vi "Remove Server.vi"(8 "error in (no error)":errorcluster, 10 "id":i32, 11 "Variant in":variant) -> (0 "error out":errorcluster, 3 "Variant out":variant)   [LabVIEW 2025, in "MCP Server.lvlib"]
doc: "Searches and removes a server from the variant lookup table. And closes it's references."
uses:
  MCP Server.lvlib
  Server Data.ctl
  Tool Data.ctl
  Input Parameter.ctl
  Output Parameter.ctl
  Logging.ctl
  User Events.ctl
  onRpc.ctl
  Prompt Data.ctl
  Prompt Argument.ctl
  resource data.ctl
  <vilib>/IlluminatedG/IG HTTP Server/HTTP Server/Server/Server.lvclass
  <vilib>/Utility/error.llb/Error Cluster From Error Code.vi
  <vilib>/ErrorRing/Error Ring.xnode
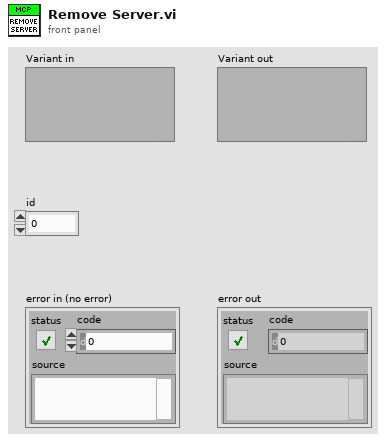
[diagram p1: front panel]
types:
  T1 = typedef "MCP Server.lvlib/Server Data.ctl" = cluster{"Name":string, "Description":string, "Tools":T2[], "Parameters":string[][], "Logging Info":T5, "User Events":T6, "Prompts":T7[], "resources":T9[], "HTTP Server":refnum<class "Server.lvclass">}
  T2 = typedef "MCP Server.lvlib/Tool Data.ctl" = cluster{"Name":string, "Description":string, "Ignored":string[], "inputs":T3[], "outputs":T4[], "VI Refnum":refnum<vi>}
  T3 = typedef "MCP Server.lvlib/Input Parameter.ctl" = cluster{"name":string, "type":string, "description":string, "required":bool, "raw name":string}
  T4 = typedef "MCP Server.lvlib/Output Parameter.ctl" = cluster{"name":string, "description":string, "type":string, "raw name":string}
  T5 = typedef "MCP Server.lvlib/Logging.ctl" = cluster{"Log":string[], "Max Length":i32}
  T6 = typedef "MCP Server.lvlib/User Events.ctl" = cluster{"onError":refnum<user-event>, "onRpc":refnum<user-event>}
  T7 = typedef "MCP Server.lvlib/Prompt Data.ctl" = cluster{"name":string, "description":string, "arguments":T8[], "return terminal name":string, "results description":string, "VI Refnum":refnum<vi>}
  T8 = typedef "MCP Server.lvlib/Prompt Argument.ctl" = cluster{"name":string, "description":string, "required":bool, "raw_name":string}
  T9 = typedef "MCP Server.lvlib/resource data.ctl" = cluster{"uri":string, "name":string, "description":string, "mimeType":string, "file path":path}
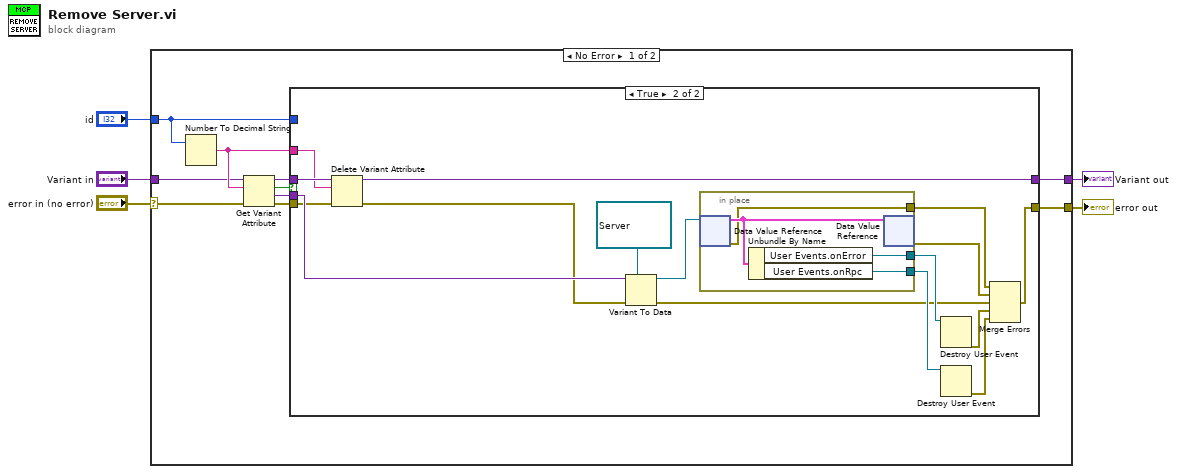
[diagram p0: block diagram]
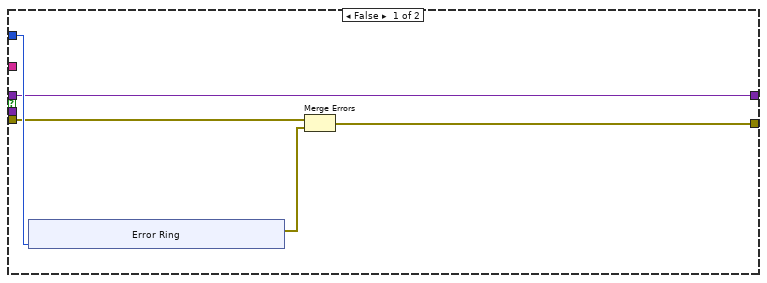
[diagram p2: hidden frame]
diagram:
  n1 = case shown="No Error" "error in (no error)" {
    selector: "error in (no error)" -> [w6 w49]
    tunnel: "id" -> [w15 _]
    tunnel: "Variant in" -> [w10 w48]
    tunnel: [w8 w49] -> w3
    tunnel: [w7 w48] -> w2
    frame No Error {
      n2 = Number To Decimal String(number=w15) -> (decimal integer string=w12:string)  [unwired: 1 in]
      n3 = Get Variant Attribute(Variant=w10, name=w12, error in=w6) -> (duplicate Variant=w11:variant, found=w14:bool, value=w13:variant, error out=w9:errorcluster)  [unwired: 1 in]
      n4 = case shown="True" w14 {
        tunnel: [w16 w43] -> w7
        tunnel: [w18 w34] -> w8
        tunnel: w9 -> [w19 w30]
        tunnel: w11 -> [w16 w42]
        tunnel: w12 -> [_ w41]
        tunnel: w13 -> [_ w40]
        tunnel: w15 -> [w20 _]
        frame False {
          n5 = xnode "Error Ring"("parameter 0"=w20) -> ("error out"=w17:errorcluster)
          n6 = Merge Errors(w19, w17) -> (w18:errorcluster)
        }
        frame True {
          n7 = Delete Variant Attribute(4:w30, 6:w41, 7:w42) -> (0:w29:errorcluster, 3:w43:variant)  [unwired: 1 out]
          n8 = Variant To Data(error in=w29, type=refnum<data-value> refnum ("data value reference"), Variant=w40) -> (data=w38:refnum<data-value>, error out=w28:errorcluster)
          n9 = in-place {
            in-place-border: [w46] -> w37
            in-place-border: [w45] -> w32
            in-place-border: [w44] -> w31
            n10 = in-place-dvr #1(w38) -> (w47:T1, w45:errorcluster)
            n11 = Unbundle By Name(w47) -> ("User Events.onError"=w46:refnum<user-event>, "User Events.onRpc"=w44:refnum<user-event>)
            n12 = in-place-dvr #1(w47) -> (w33:errorcluster)  [unwired: 1 out]
          }
          n13 = Destroy User Event(user event=w37) -> (error out=w36:errorcluster)  [unwired: 1 in]
          n14 = Destroy User Event(user event=w31) -> (error out=w35:errorcluster)  [unwired: 1 in]
          n15 = Merge Errors(w32, w33, w28, w36, w35) -> (w34:errorcluster)
        }
      }
    }
    frame Error {
    }
  }
  "error out" <- w3
  "Variant out" <- w2
